vi "Calibration Helper.vi"(6 "Std Devs":cluster{"H":dbl, "S":dbl, "V":dbl}={"H"=4.0, "S"=6.0, "V"=4.0}, 7 "Color Display":refnum<vi>, 8 "Color Mode":u16(ring)=2 items=["RGB", "HSL", "HSV", "HSI", "CIE L*a*b*", "CIE XYZ"], 10 "Image":T1, 11 "Image Ctl Refnum":refnum<vi>) -> (2 "Changed":bool)   [LabVIEW 2015]
uses:
  <vilib>/vision/Image Controls.llb/IMAQ Image.ctl
  <vilib>/vision/NI_Vision_Development_Module.lvlib
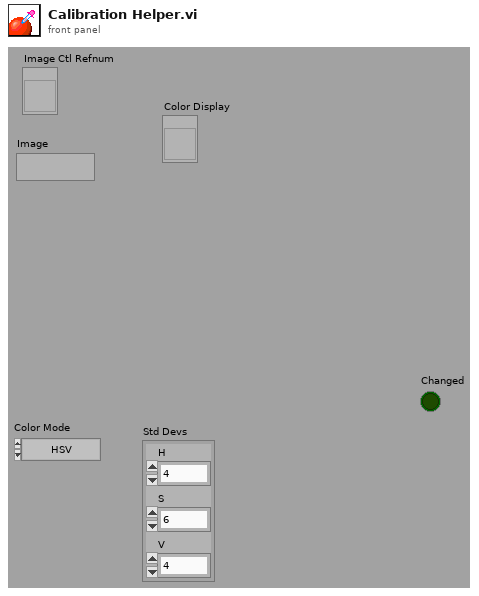
[diagram p1: front panel]
types:
  T1 = typedef "IMAQ Image.ctl" = refnum<image>
  T2 = typedef "Image Type" = u32
  T3 = cluster{"Global Rectangle":i32[], "Contours":cluster{"Contour Type":u32, "ROI Type":u32, "Points":i32[]}[]}
  T4 = cluster{"histogram":u32[], "Minimal Value":sgl, "Maximal Value":sgl, "Starting Value":sgl, "Interval Width":sgl, "Mean Value":sgl, "Standard  Variation":sgl, "Area (pixels)":i32}
  T5 = cluster{"histogram":u32[], "Minimal Value":sgl, "Maximal Value":sgl, "Starting Value":sgl, "Interval Width":sgl, "Mean Value":sgl, "Standard  Variation":sgl, "Area (pixels)":i32}[]
  T6 = cluster{"[0]":cluster{dbl, dbl}, "[1]":cluster{dbl, dbl}, "[2]":cluster{dbl, dbl}}
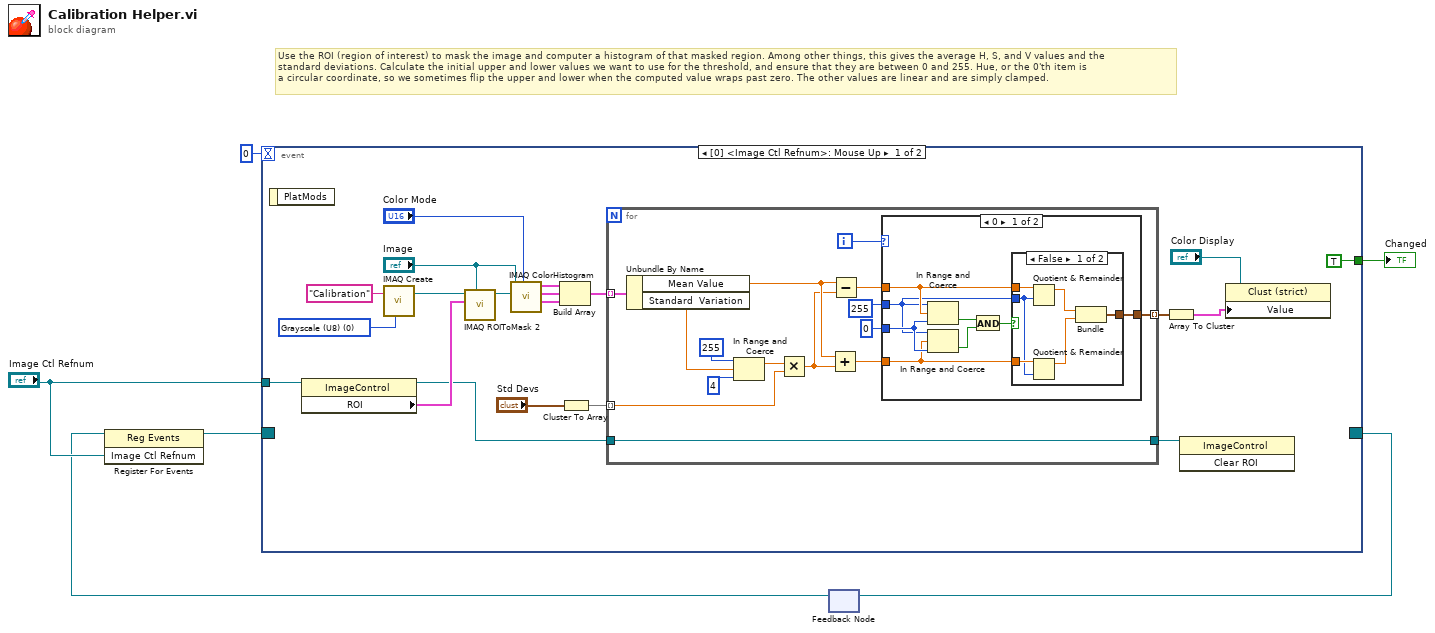
[diagram p0: block diagram]
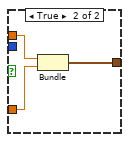
[diagram p2: hidden frame]
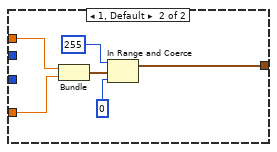
[diagram p3: hidden frame]
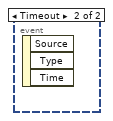
[diagram p4: hidden frame]
diagram:
  # "Use the ROI (region of interest) to mask the image and computer a histogram of that masked region. Among other things, this gives the average H, S, and V values and the\nstandard deviations. Calculate the initial upper and lower values we want to use for the threshold, and ensure that they are between 0 and 255. Hue, or the 0'th item is\na circular coordinate, so we sometimes flip the upper and lower when the computed value wraps past zero. The other values are linear and are simply clamped."
  n1 = feedback #1() -> (w2:refnum<event-registration>)  [unwired: 1 in]
  n2 = register-events(reference=w2, "Image Ctl Refnum") -> (reference out=w4:refnum<event-registration>)  [unwired: 1 in, 1 out]
  n3 = event shown="[0] <Image Ctl Refnum>: Mouse Up" {
    selector: w4 -> [_ _]
    dyn-events: [_ _] -> w3
    timeout: 0 -> [_ _]
    tunnel: "Image Ctl Refnum" -> [w13 _]
    tunnel: [TRUE _] -> w1
    event Mouse Up {
      w26 = T2 0 items=["Grayscale (U8)", "Grayscale (I16)", "Grayscale (SGL)", "Complex (CSG)", "RGB (U32)", "HSL (U32)", "RGB (U64)", "Grayscale (U16)"] ("Image Type")
      n4 = event-data() -> ()  [unwired: 1 in, 1 out]
      n5 = property on="Property Node" class="ImageControl"(reference=w13) -> (reference out=w10:refnum<vi>, "ROI"=w12:T3)  [unwired: 1 in, 1 out]
      n6 = call "IMAQ Create"("Image Name"="Calibration", "Image Type"=w26) -> ("New Image"=w23:T1)  [unwired: 3 in, 1 out]
      n7 = call "IMAQ ROIToMask 2"("Image Model"="Image", "ROI Descriptor"=w12, "Image"=w23) -> ("Image Out"=w24:T1)  [unwired: 6 in, 2 out]
      n8 = call "IMAQ ColorHistogram"("Color Mode"="Color Mode", "Image Src"="Image", "Image Mask"=w24) -> ("Red or Hue or X or L* Histogram Report"=w19:T4, "Green or Sat or Y or a* Histogram Report"=w18:T4, "Blue or Luma or Val or Inten or Z or b* Histogram Report"=w17:T4)  [unwired: 3 in, 1 out]
      n9 = Build Array(w19, w18, w17) -> (w15:T5)
      n10 = Cluster To Array(cluster="Std Devs") -> (array=w16:dbl[])
      n11 = for {
        tunnel: w16 -> [w37] mode=indexing
        tunnel: w15 -> [w41] mode=indexing
        tunnel: [w32] -> w14 mode=indexing
        tunnel: [w27] -> w11
        tunnel: w10 -> [w27]
        i -> [w30]
        n12 = Unbundle By Name(w41) -> ("Mean Value"=w35:sgl, "Standard  Variation"=w38:sgl)
        n13 = In Range and Coerce(upper limit=255, x=w38, lower limit=4) -> (coerced(x)=w36:sgl)  [unwired: 1 out]
        n14 = Multiply(x=w36, y=w37) -> (x*y=w31:dbl)
        n15 = Add(x=w35, y=w31) -> (x+y=w33:dbl)
        n16 = Subtract(x=w35, y=w31) -> (x-y=w34:dbl)
        n17 = case shown="0" w30 {
          tunnel: w34 -> [w44 w61]
          tunnel: w33 -> [w43 w60]
          tunnel: [w46 w59] -> w32
          tunnel: 255 -> [w42 _]
          tunnel: 0 -> [w45 _]
          frame 0 {
            n18 = In Range and Coerce(upper limit=w42, x=w44, lower limit=w45) -> (In Range?=w48:bool)  [unwired: 1 out]
            n19 = In Range and Coerce(upper limit=w42, x=w43, lower limit=w45) -> (In Range?=w47:bool)  [unwired: 1 out]
            n20 = And(x=w48, y=w47) -> (x .and. y?=w49:bool)
            n21 = case shown="False" w49 {
              tunnel: [w52 w58] -> w46
              tunnel: w44 -> [w55 w56]
              tunnel: w43 -> [w54 w57]
              tunnel: w42 -> [w53 _]
              frame False {
                n22 = Quotient & Remainder(x=w55, y=w53) -> (x-y*floor(x/y)=w50:dbl)  [unwired: 1 out]
                n23 = Quotient & Remainder(x=w54, y=w53) -> (x-y*floor(x/y)=w51:dbl)  [unwired: 1 out]
                n24 = Bundle(w50, w51) -> (w52:cluster{dbl, dbl})  [unwired: 1 in]
              }
              frame True {
                n25 = Bundle(w56, w57) -> (w58:cluster{dbl, dbl})  [unwired: 1 in]
              }
            }
          }
          frame 1, Default {
            n26 = Bundle(w61, w60) -> (w64:cluster{dbl, dbl})  [unwired: 1 in]
            n27 = In Range and Coerce(upper limit=255, x=w64, lower limit=0) -> (coerced(x)=w59:cluster{dbl, dbl})  [unwired: 1 out]
          }
        }
      }
      n28 = Array To Cluster(array=w14) -> (cluster=w7:T6)
      n29 = invoke on="Invoke Node" class="ImageControl" method="Clear ROI"(reference=w11) -> ()  [unwired: 2 in, 3 out]
      n30 = property class="Clust (strict)"(reference="Color Display", "Value"=w7) -> ()  [unwired: 1 in, 2 out]
    }
    event Timeout {
      n31 = event-data() -> ()  [unwired: 1 in, 3 out]
    }
  }
  "Changed" <- w1
  n32 = feedback-in #1(w3) -> ()
